vi "16DUT Plot Subvi.vi"(6 "No of Rows":u64=10496, 7 "Plot":T1(ring), 8 "error in (no error)":errorcluster, 10 "Input T0":string[][](table), 11 "Input":string[][](table)) -> (0 "error out":errorcluster, 3 "Delta C_Min Plot":dbl[][](graph) caption="(Y) Multi Plot 2")   [LabVIEW 2012]
panel:
  in  "Start":bool=TRUE
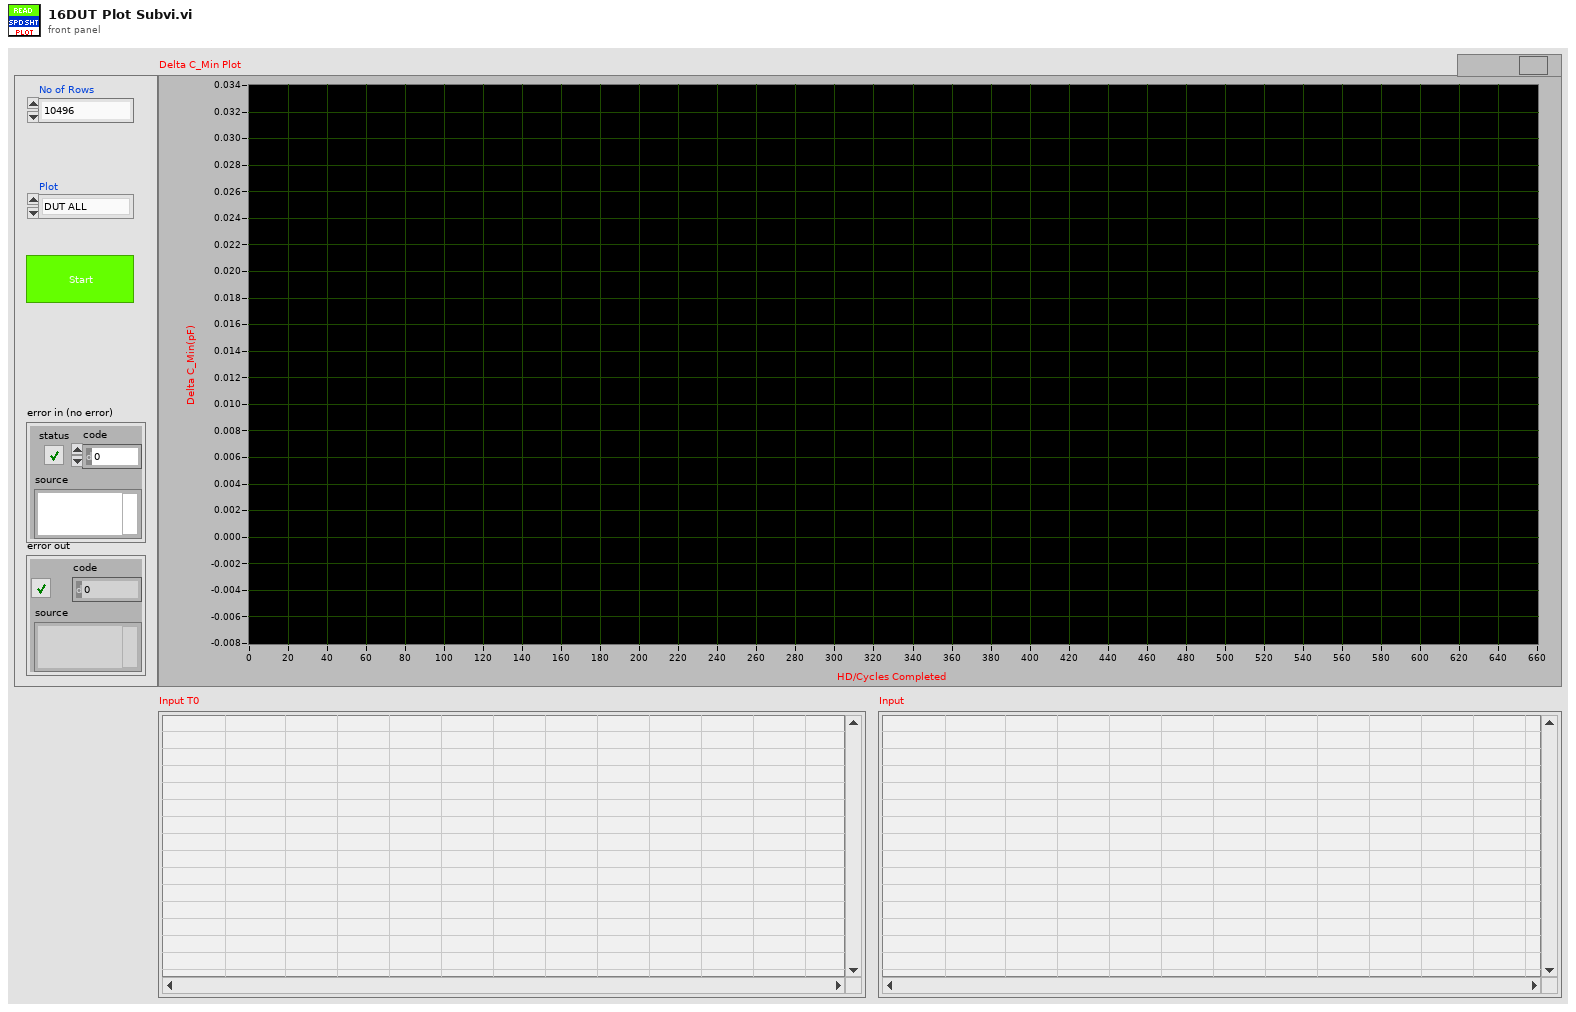
[diagram p1: front panel]
types:
  T1 = enum16{"DUT ALL", "DUT 01", "DUT 02", "DUT 03", "DUT 04", "DUT 05", "DUT 06", "DUT 07", "DUT 08", "DUT 09", "DUT 10", "DUT 11", "DUT 12", "DUT 13", "DUT 14", "DUT 15", "DUT 16"}
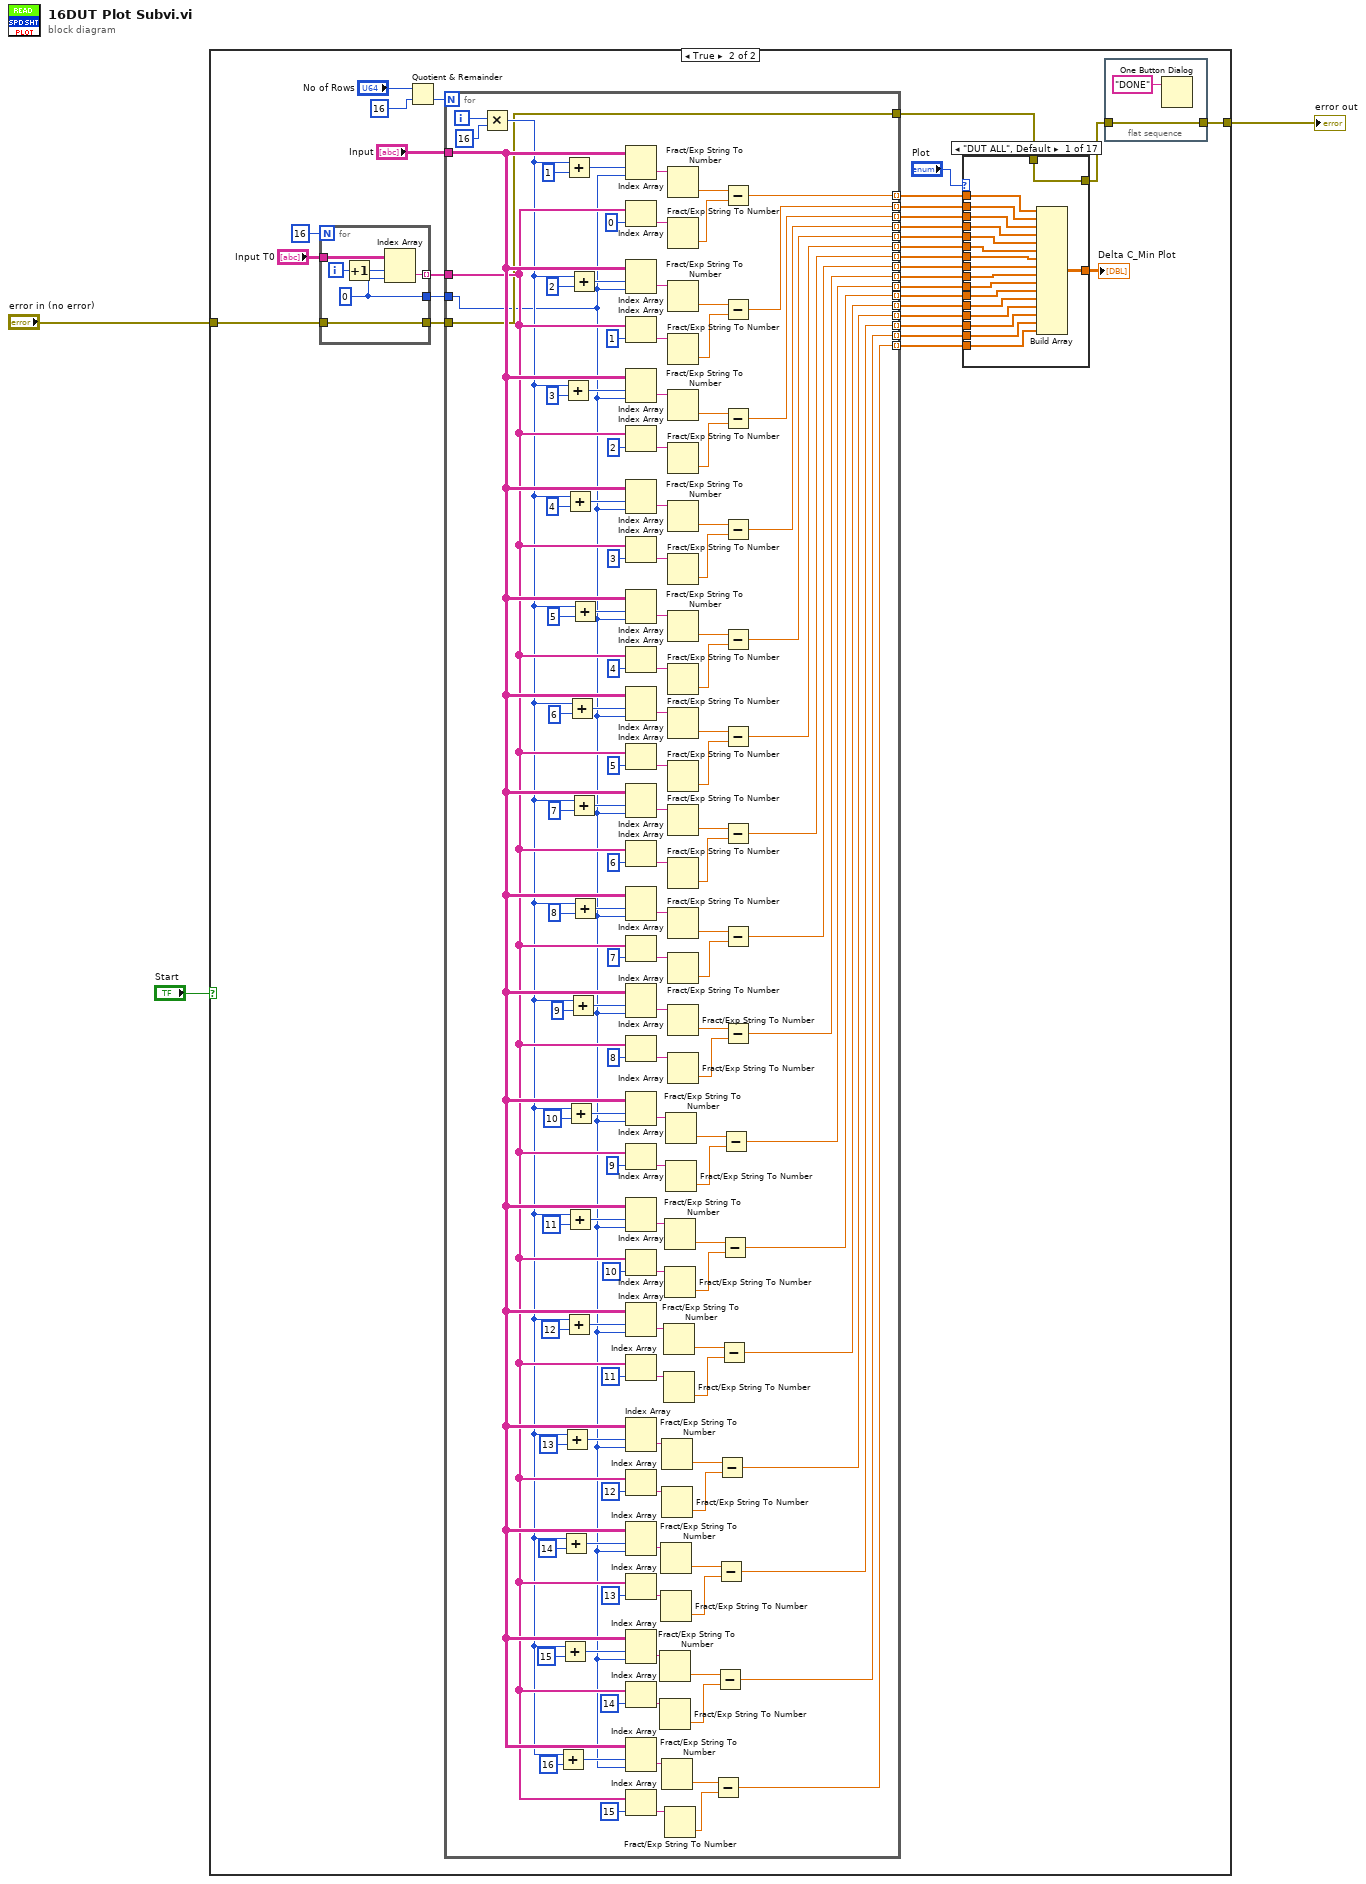
[diagram p0: block diagram]
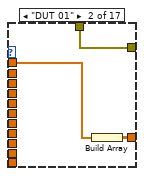
[diagram p3: hidden frame]
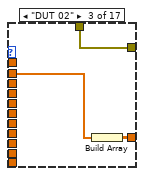
[diagram p4: hidden frame]
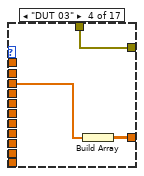
[diagram p5: hidden frame]
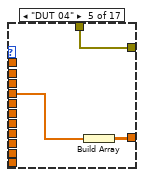
[diagram p6: hidden frame]
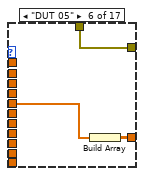
[diagram p7: hidden frame]
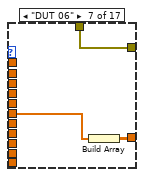
[diagram p8: hidden frame]
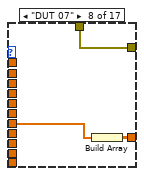
[diagram p9: hidden frame]
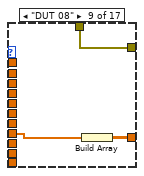
[diagram p10: hidden frame]
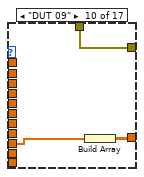
[diagram p11: hidden frame]
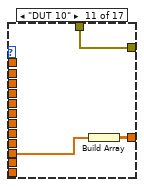
[diagram p12: hidden frame]
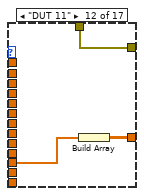
[diagram p13: hidden frame]
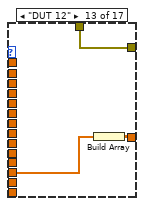
[diagram p14: hidden frame]
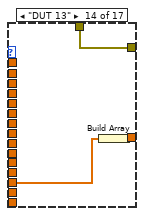
[diagram p15: hidden frame]
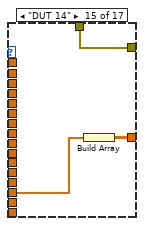
[diagram p16: hidden frame]
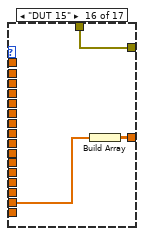
[diagram p17: hidden frame]
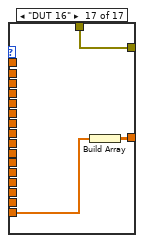
[diagram p18: hidden frame]
diagram:
  n1 = case shown="True" "Start" {
    tunnel: "error in (no error)" -> [w4 w7]
    tunnel: [w4 w9] -> w2
    frame False {
    }
    frame True {
      n2 = for {
        N: 16 -> [_]
        tunnel: "Input T0" -> [w244]
        tunnel: [w243] -> w34 mode=indexing
        tunnel: [w240] -> w12
        tunnel: w7 -> [w240]
        tunnel: [w239] -> w6
        i -> [w242]
        w239 = 0 ("disabled index (col)")
        n3 = Increment(x=w242) -> (x+1=w241:i32)
        n4 = Index Array(array=w244, index (row)=w241, index (col)=w239) -> (element=w243:string)
      }
      n5 = Quotient & Remainder(x="No of Rows", y=16) -> (floor(x/y)=w31:u64)  [unwired: 1 out]
      n6 = for {
        N: w31 -> [_]
        tunnel: "Input" -> [w125]
        tunnel: w34 -> [w124]
        tunnel: [w122] -> w29 mode=indexing
        tunnel: [w121] -> w28 mode=indexing
        tunnel: [w120] -> w27 mode=indexing
        tunnel: [w119] -> w26 mode=indexing
        tunnel: [w118] -> w25 mode=indexing
        tunnel: [w117] -> w24 mode=indexing
        tunnel: [w116] -> w23 mode=indexing
        tunnel: [w115] -> w22 mode=indexing
        tunnel: [w114] -> w21 mode=indexing
        tunnel: [w113] -> w20 mode=indexing
        tunnel: [w112] -> w19 mode=indexing
        tunnel: [w111] -> w18 mode=indexing
        tunnel: [w110] -> w17 mode=indexing
        tunnel: [w109] -> w16 mode=indexing
        tunnel: [w108] -> w15 mode=indexing
        tunnel: [w107] -> w14 mode=indexing
        tunnel: w12 -> [w106]
        tunnel: [w106] -> w11
        tunnel: w6 -> [w104]
        i -> [w105]
        n7 = Multiply(x=w105, y=16) -> (x*y=w123:i32)
        n8 = Add(x=w123, y=16) -> (x+y=w130:i32)
        n9 = Add(x=w123, y=15) -> (x+y=w135:i32)
        n10 = Add(x=w123, y=14) -> (x+y=w144:i32)
        n11 = Add(x=w123, y=13) -> (x+y=w149:i32)
        n12 = Add(x=w123, y=3) -> (x+y=w204:i32)
        n13 = Add(x=w123, y=1) -> (x+y=w226:i32)
        n14 = Add(x=w123, y=12) -> (x+y=w158:i32)
        n15 = Add(x=w123, y=4) -> (x+y=w203:i32)
        n16 = Add(x=w123, y=11) -> (x+y=w163:i32)
        n17 = Add(x=w123, y=10) -> (x+y=w172:i32)
        n18 = Add(x=w123, y=6) -> (x+y=w189:i32)
        n19 = Add(x=w123, y=9) -> (x+y=w219:i32)
        n20 = Add(x=w123, y=2) -> (x+y=w223:i32)
        n21 = Add(x=w123, y=7) -> (x+y=w182:i32)
        n22 = Add(x=w123, y=5) -> (x+y=w196:i32)
        n23 = Add(x=w123, y=8) -> (x+y=w176:i32)
        n24 = Index Array(array=w125, index (row)=w226, index (col)=w104) -> (element=w237:string)
        n25 = Index Array(array=w124, index=0) -> (element=w235:string)
        n26 = Index Array(array=w125, index (row)=w223, index (col)=w104) -> (element=w228:string)
        n27 = Index Array(array=w124, index=1) -> (element=w230:string)
        n28 = Index Array(array=w125, index (row)=w204, index (col)=w104) -> (element=w216:string)
        n29 = Index Array(array=w124, index=2) -> (element=w214:string)
        n30 = Index Array(array=w125, index (row)=w203, index (col)=w104) -> (element=w206:string)
        n31 = Index Array(array=w124, index=3) -> (element=w208:string)
        n32 = Index Array(array=w125, index (row)=w196, index (col)=w104) -> (element=w202:string)
        n33 = Index Array(array=w124, index=4) -> (element=w200:string)
        n34 = Index Array(array=w125, index (row)=w189, index (col)=w104) -> (element=w191:string)
        n35 = Index Array(array=w124, index=5) -> (element=w193:string)
        n36 = Index Array(array=w125, index (row)=w182, index (col)=w104) -> (element=w188:string)
        n37 = Index Array(array=w124, index=6) -> (element=w186:string)
        n38 = Index Array(array=w125, index (row)=w176, index (col)=w104) -> (element=w175:string)
        n39 = Index Array(array=w124, index=7) -> (element=w179:string)
        n40 = Index Array(array=w125, index (row)=w219, index (col)=w104) -> (element=w222:string)
        n41 = Index Array(array=w124, index=8) -> (element=w220:string)
        n42 = Index Array(array=w125, index (row)=w172, index (col)=w104) -> (element=w169:string)
        n43 = Index Array(array=w124, index=9) -> (element=w171:string)
        n44 = Index Array(array=w125, index (row)=w163, index (col)=w104) -> (element=w166:string)
        n45 = Index Array(array=w124, index=10) -> (element=w164:string)
        n46 = Index Array(array=w125, index (row)=w158, index (col)=w104) -> (element=w155:string)
        n47 = Index Array(array=w124, index=11) -> (element=w157:string)
        n48 = Index Array(array=w125, index (row)=w149, index (col)=w104) -> (element=w152:string)
        n49 = Index Array(array=w124, index=12) -> (element=w150:string)
        n50 = Index Array(array=w125, index (row)=w144, index (col)=w104) -> (element=w141:string)
        n51 = Index Array(array=w124, index=13) -> (element=w143:string)
        n52 = Index Array(array=w125, index (row)=w135, index (col)=w104) -> (element=w138:string)
        n53 = Index Array(array=w124, index=14) -> (element=w136:string)
        n54 = Index Array(array=w125, index (row)=w130, index (col)=w104) -> (element=w127:string)
        n55 = Index Array(array=w124, index=15) -> (element=w129:string)
        n56 = Fract/Exp String To Number(string=w138) -> (number=w134:dbl)  [unwired: 3 in, 1 out]
        n57 = Fract/Exp String To Number(string=w136) -> (number=w133:dbl)  [unwired: 3 in, 1 out]
        n58 = Fract/Exp String To Number(string=w141) -> (number=w145:dbl)  [unwired: 3 in, 1 out]
        n59 = Fract/Exp String To Number(string=w143) -> (number=w146:dbl)  [unwired: 3 in, 1 out]
        n60 = Fract/Exp String To Number(string=w152) -> (number=w148:dbl)  [unwired: 3 in, 1 out]
        n61 = Fract/Exp String To Number(string=w150) -> (number=w147:dbl)  [unwired: 3 in, 1 out]
        n62 = Fract/Exp String To Number(string=w127) -> (number=w131:dbl)  [unwired: 3 in, 1 out]
        n63 = Fract/Exp String To Number(string=w155) -> (number=w159:dbl)  [unwired: 3 in, 1 out]
        n64 = Fract/Exp String To Number(string=w157) -> (number=w160:dbl)  [unwired: 3 in, 1 out]
        n65 = Fract/Exp String To Number(string=w166) -> (number=w162:dbl)  [unwired: 3 in, 1 out]
        n66 = Fract/Exp String To Number(string=w164) -> (number=w161:dbl)  [unwired: 3 in, 1 out]
        n67 = Fract/Exp String To Number(string=w129) -> (number=w132:dbl)  [unwired: 3 in, 1 out]
        n68 = Fract/Exp String To Number(string=w169) -> (number=w173:dbl)  [unwired: 3 in, 1 out]
        n69 = Fract/Exp String To Number(string=w171) -> (number=w174:dbl)  [unwired: 3 in, 1 out]
        n70 = Fract/Exp String To Number(string=w237) -> (number=w234:dbl)  [unwired: 3 in, 1 out]
        n71 = Fract/Exp String To Number(string=w235) -> (number=w233:dbl)  [unwired: 3 in, 1 out]
        n72 = Fract/Exp String To Number(string=w228) -> (number=w231:dbl)  [unwired: 3 in, 1 out]
        n73 = Fract/Exp String To Number(string=w230) -> (number=w232:dbl)  [unwired: 3 in, 1 out]
        n74 = Fract/Exp String To Number(string=w216) -> (number=w213:dbl)  [unwired: 3 in, 1 out]
        n75 = Fract/Exp String To Number(string=w214) -> (number=w212:dbl)  [unwired: 3 in, 1 out]
        n76 = Fract/Exp String To Number(string=w206) -> (number=w209:dbl)  [unwired: 3 in, 1 out]
        n77 = Fract/Exp String To Number(string=w208) -> (number=w210:dbl)  [unwired: 3 in, 1 out]
        n78 = Fract/Exp String To Number(string=w202) -> (number=w199:dbl)  [unwired: 3 in, 1 out]
        n79 = Fract/Exp String To Number(string=w200) -> (number=w198:dbl)  [unwired: 3 in, 1 out]
        n80 = Fract/Exp String To Number(string=w191) -> (number=w194:dbl)  [unwired: 3 in, 1 out]
        n81 = Fract/Exp String To Number(string=w193) -> (number=w195:dbl)  [unwired: 3 in, 1 out]
        n82 = Fract/Exp String To Number(string=w188) -> (number=w185:dbl)  [unwired: 3 in, 1 out]
        n83 = Fract/Exp String To Number(string=w186) -> (number=w184:dbl)  [unwired: 3 in, 1 out]
        n84 = Fract/Exp String To Number(string=w175) -> (number=w180:dbl)  [unwired: 3 in, 1 out]
        n85 = Fract/Exp String To Number(string=w179) -> (number=w181:dbl)  [unwired: 3 in, 1 out]
        n86 = Fract/Exp String To Number(string=w222) -> (number=w218:dbl)  [unwired: 3 in, 1 out]
        n87 = Fract/Exp String To Number(string=w220) -> (number=w217:dbl)  [unwired: 3 in, 1 out]
        n88 = Subtract(x=w131, y=w132) -> (x-y=w107:dbl)
        n89 = Subtract(x=w134, y=w133) -> (x-y=w108:dbl)
        n90 = Subtract(x=w145, y=w146) -> (x-y=w109:dbl)
        n91 = Subtract(x=w148, y=w147) -> (x-y=w110:dbl)
        n92 = Subtract(x=w159, y=w160) -> (x-y=w111:dbl)
        n93 = Subtract(x=w162, y=w161) -> (x-y=w112:dbl)
        n94 = Subtract(x=w173, y=w174) -> (x-y=w113:dbl)
        n95 = Subtract(x=w234, y=w233) -> (x-y=w122:dbl)
        n96 = Subtract(x=w231, y=w232) -> (x-y=w121:dbl)
        n97 = Subtract(x=w213, y=w212) -> (x-y=w120:dbl)
        n98 = Subtract(x=w209, y=w210) -> (x-y=w119:dbl)
        n99 = Subtract(x=w199, y=w198) -> (x-y=w118:dbl)
        n100 = Subtract(x=w194, y=w195) -> (x-y=w117:dbl)
        n101 = Subtract(x=w185, y=w184) -> (x-y=w116:dbl)
        n102 = Subtract(x=w180, y=w181) -> (x-y=w115:dbl)
        n103 = Subtract(x=w218, y=w217) -> (x-y=w114:dbl)
      }
      n104 = case shown="\"DUT ALL\", Default" "Plot" {
        tunnel: w29 -> [w55 w58 _ _ _ _ _ _ _ _ _ _ _ _ _ _ _]
        tunnel: w28 -> [w54 _ w60 _ _ _ _ _ _ _ _ _ _ _ _ _ _]
        tunnel: w27 -> [w53 _ _ w64 _ _ _ _ _ _ _ _ _ _ _ _ _]
        tunnel: w26 -> [w52 _ _ _ w66 _ _ _ _ _ _ _ _ _ _ _ _]
        tunnel: w25 -> [w51 _ _ _ _ w70 _ _ _ _ _ _ _ _ _ _ _]
        tunnel: w24 -> [w50 _ _ _ _ _ w72 _ _ _ _ _ _ _ _ _ _]
        tunnel: w23 -> [w49 _ _ _ _ _ _ w75 _ _ _ _ _ _ _ _ _]
        tunnel: w22 -> [w48 _ _ _ _ _ _ _ w79 _ _ _ _ _ _ _ _]
        tunnel: w21 -> [w47 _ _ _ _ _ _ _ _ w82 _ _ _ _ _ _ _]
        tunnel: w20 -> [w46 _ _ _ _ _ _ _ _ _ w85 _ _ _ _ _ _]
        tunnel: w19 -> [w45 _ _ _ _ _ _ _ _ _ _ w88 _ _ _ _ _]
        tunnel: w18 -> [w44 _ _ _ _ _ _ _ _ _ _ _ w91 _ _ _ _]
        tunnel: w17 -> [w43 _ _ _ _ _ _ _ _ _ _ _ _ w94 _ _ _]
        tunnel: w16 -> [w42 _ _ _ _ _ _ _ _ _ _ _ _ _ w97 _ _]
        tunnel: w15 -> [w41 _ _ _ _ _ _ _ _ _ _ _ _ _ _ w100 _]
        tunnel: w14 -> [w40 _ _ _ _ _ _ _ _ _ _ _ _ _ _ _ w102]
        tunnel: [w39 w57 w61 w63 w67 w69 w73 w76 w78 w81 w84 w87 w90 w93 w96 w99 w103] -> w13
        tunnel: w11 -> [w38 w56 w59 w62 w65 w68 w71 w74 w77 w80 w83 w86 w89 w92 w95 w98 w101]
        tunnel: [w38 w56 w59 w62 w65 w68 w71 w74 w77 w80 w83 w86 w89 w92 w95 w98 w101] -> w10
        frame "DUT ALL", Default {
          n105 = Build Array(w55, w54, w53, w52, w51, w50, w49, w48, w47, w46, w45, w44, w43, w42, w41, w40) -> (w39:dbl[][])
        }
        frame "DUT 01" {
          n106 = Build Array(w58) -> (w57:dbl[][])
        }
        frame "DUT 02" {
          n107 = Build Array(w60) -> (w61:dbl[][])
        }
        frame "DUT 03" {
          n108 = Build Array(w64) -> (w63:dbl[][])
        }
        frame "DUT 04" {
          n109 = Build Array(w66) -> (w67:dbl[][])
        }
        frame "DUT 05" {
          n110 = Build Array(w70) -> (w69:dbl[][])
        }
        frame "DUT 06" {
          n111 = Build Array(w72) -> (w73:dbl[][])
        }
        frame "DUT 07" {
          n112 = Build Array(w75) -> (w76:dbl[][])
        }
        frame "DUT 08" {
          n113 = Build Array(w79) -> (w78:dbl[][])
        }
        frame "DUT 09" {
          n114 = Build Array(w82) -> (w81:dbl[][])
        }
        frame "DUT 10" {
          n115 = Build Array(w85) -> (w84:dbl[][])
        }
        frame "DUT 11" {
          n116 = Build Array(w88) -> (w87:dbl[][])
        }
        frame "DUT 12" {
          n117 = Build Array(w91) -> (w90:dbl[][])
        }
        frame "DUT 13" {
          n118 = Build Array(w94) -> (w93:dbl[][])
        }
        frame "DUT 14" {
          n119 = Build Array(w97) -> (w96:dbl[][])
        }
        frame "DUT 15" {
          n120 = Build Array(w100) -> (w99:dbl[][])
        }
        frame "DUT 16" {
          n121 = Build Array(w102) -> (w103:dbl[][])
        }
      }
      "Delta C_Min Plot" <- w13
      n122 = flat-sequence {
        tunnel: w10 -> [w36]
        tunnel: [w36] -> w9
        frame #0 {
          n123 = One Button Dialog(message="DONE") -> ()  [unwired: 1 in, 1 out]
        }
      }
    }
  }
  "error out" <- w2
